vi "LoadActor.vi"(8 "error in (no error)":errorcluster, 9 "CameraTestingUI":refnum<class "CameraTestingUI.lvclass">, 10 "Connection String":string, 11 "ICamera in":refnum<class "ICamera.lvclass">) -> (0 "error out":errorcluster)   [LabVIEW 2020, in "CameraTesting.lvlib" / "CameraTesting.lvclass"]
uses:
  CameraTesting.lvclass
  CameraTesting.lvclass/CameraTesting.ctl
  <vilib>/ActorFramework/Actor/Actor.lvclass
  CameraTesting Messages/Init Msg/Init Msg.lvclass
  <vilib>/ActorFramework/Message Enqueuer/Message Priority.ctl
  <vilib>/ActorFramework/Message Enqueuer/Message Enqueuer.lvclass
  C:/Program Files (x86)/National Instruments/LabVIEW 2020/vi.lib/ActorFramework/Actor/Actor.lvclass
  E:/GitHub/Evaluation_Test/Labview/src/CameraTestingApp/CameraTesting/CameraTesting/CameraTesting.lvclass
  E:/GitHub/Evaluation_Test/Labview/src/CameraTestingApp/ICameraTesting/ICameraTesting/ICameraTesting.lvclass
  CameraTestingUI/CameraTestingUI/CameraTestingUI.lvclass
  E:/GitHub/Evaluation_Test/Labview/src/CameraTestingApp/CameraTestingUI/CameraTestingUI/CameraTestingUI.lvclass
  E:/GitHub/Evaluation_Test/Labview/src/CameraTestingApp/ICameraTestingUI/ICameraTestingUI/ICameraTestingUI.lvclass
  Camera/ICamera/ICamera/ICamera.lvclass
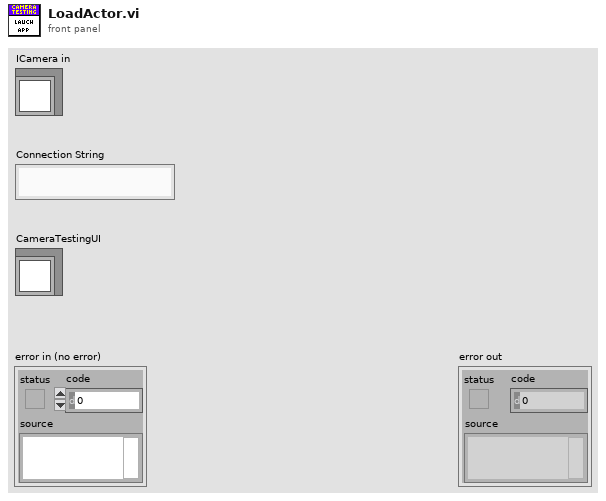
[diagram p1: front panel]
types:
  T1 = typedef "Actor Framework.lvlib/Message Enqueuer.lvclass/Message Priority.ctl" = enum16{"Low", "Normal", "High"}
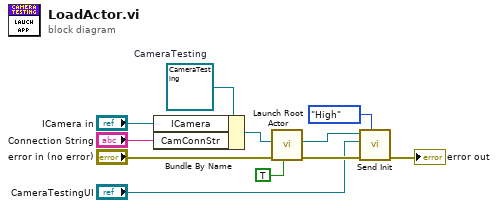
[diagram p0: block diagram]
diagram:
  w6 = refnum<class "CameraTesting.lvclass"> refnum  # CameraTesting
  n1 = Bundle By Name(cluster=w6, "ICamera"="ICamera in", "CamConnStr"="Connection String") -> (w5:refnum<class "CameraTesting.lvclass">)
  n2 = call <vilib>:"Launch Root Actor.vi"("Open Actor Core front panel? (F)"=TRUE, "error in (no error)"="error in (no error)", "Actor"=w5) -> ("error out"=w10:errorcluster, "Actor's Enqueuer"=w11:refnum<class "Message Enqueuer.lvclass">)  [unwired: 7 in]
  n3 = call "Send Init.vi"("Message Priority (Normal)"=Message_Priority."High", "error in (no error)"=w10, "ICameraTestingUI.lvlib:ICameraTestingUI.lvclass"="CameraTestingUI", "Message Enqueuer"=w11) -> ("error out"=→"error out":errorcluster)  [unwired: 6 in, 1 out]
